vi "SEQ Get.vi"(8 "error in (no error)":errorcluster, 11 "Data Refnum":T1) -> (0 "error out":errorcluster, 2 "dummy":bool, 3 "Data Refnum out":T1)   [LabVIEW 2009]
doc: "This is a template VI for the SEQ Get function. It is not used in the course because the Set and Get are created with a different method that leverages scripting. \n\nAAL 9/09"
uses:
  Controls/SEQ DataRef.ctl
  Controls/SEQ Data.ctl
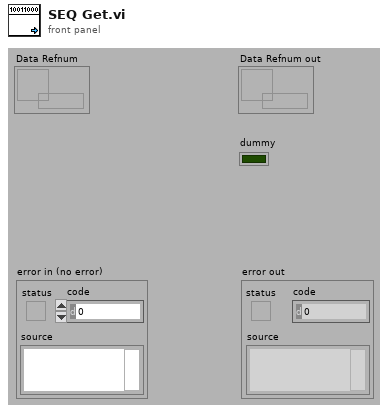
[diagram p1: front panel]
types:
  T1 = typedef "SEQ DataRef.ctl" = refnum<queue>
  T2 = typedef "SEQ Data.ctl" = cluster{"Numeric":dbl}
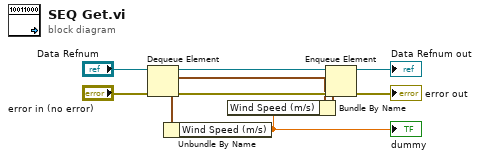
[diagram p0: block diagram]
diagram:
  n1 = Dequeue Element(queue="Data Refnum", error in (no error)="error in (no error)") -> (queue out=w3:T1, element=w2:T2, error out=w4:errorcluster)  [unwired: 2 out]
  n2 = Unbundle By Name(w2) -> ("Wind Speed (m/s)"=w8:dbl)
  "dummy" <- w8
  n3 = Bundle By Name(cluster=w2, "Wind Speed (m/s)"=w8) -> (w1:T2)
  n4 = Enqueue Element(queue=w3, element=w1, error in (no error)=w4) -> (queue out=→"Data Refnum out":T1, error out=→"error out":errorcluster)  [unwired: 2 out]
